vi "meas02a.vi"() -> ()   [LabVIEW 2015]
uses:
  <vilib>/DAQmx/write.llb/DAQmx Write (Analog Wfm 1Chan NSamp).vi
  <vilib>/DAQmx/create/channels.llb/DAQmx Create Channel (AO-Voltage-Basic).vi
  <vilib>/DAQmx/configure/timing.llb/DAQmx Timing (Sample Clock).vi
  <vilib>/measure/macond.llb/FIR Filter for 1 Chan.vi
  <vilib>/DAQmx/miscellaneous.llb/DAQmx Fill In Error Info.vi
  <vilib>/DAQmx/create/channels.llb/DAQmx Create Channel (CO-Pulse Generation-Frequency).vi
  <vilib>/DAQmx/configure/timing.llb/DAQmx Timing (Implicit).vi
  <vilib>/Utility/file.llb/Write Delimited Spreadsheet (DBL).vi
  <vilib>/measure/NI_MABase.lvlib
  <vilib>/measure/NI_MAPro.lvlib
panel:
  in  "Vertical Coupling (1: DC)":i32(ring)=1 items=["AC", "DC", "Ground"]
  out "Waveform Data":waveform(dbl)(graph)
  out "Log-Log Frequency and Gain":cluster{"Y":dbl[], "Y":dbl[]}[](graph)
  out "freq in":dbl
  out "Loop #":i32
  out "detected amplitude":dbl format="%.2p"
  out "detected frequency":dbl format="%.2p"
  in  "Trigger Level (0.0 V)":dbl
  in  "Trigger Mode (0: Auto)":i32(ring) items=["Auto", "Normal"]
  in  "VISA resource name":refnum<visa-resource-name>
  in  "# Points":dbl
  in  "Highest Freq":dbl
  in  "Lowest Freq":dbl
  in  "Frequency (Hz)":dbl
  in  "Stop Clock":bool
  in  "Run":bool
  in  "stop":bool
  in  "physical channels":tag
  out "Amplitude":dbl
  in  "Amplitude":dbl(knob) scale=0.0..5.0
  in  "signal type":T1(ring)
  # "Clock"
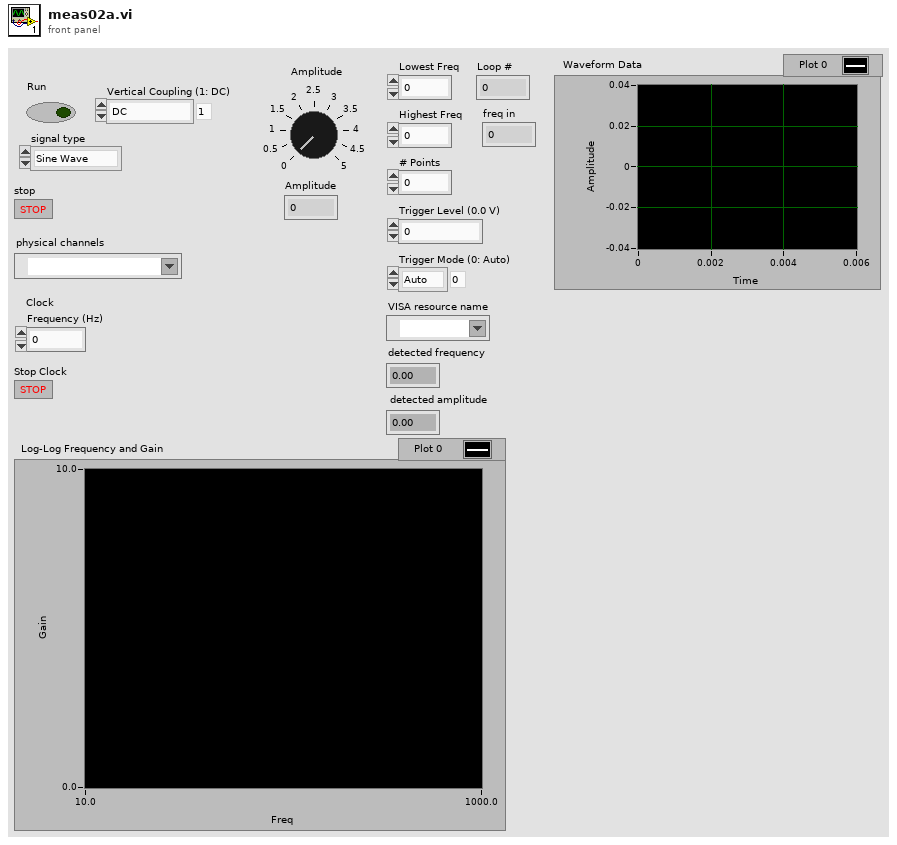
[diagram p1: front panel]
types:
  T1 = enum16{"Sine Wave", "Triangle Wave", "Square Wave", "Sawtooth Wave"}
  T2 = cluster{"Topology":enum16{"Off", "FIR by Specification", "Equi-ripple FIR", "Windowed FIR"}, "Type":enum16{"Lowpass", "Highpass", "Bandpass", "Bandstop"}, "#Taps":i32, "Lower PB":dbl, "Upper PB":dbl, "Lower SB":dbl, "Upper SB":dbl}
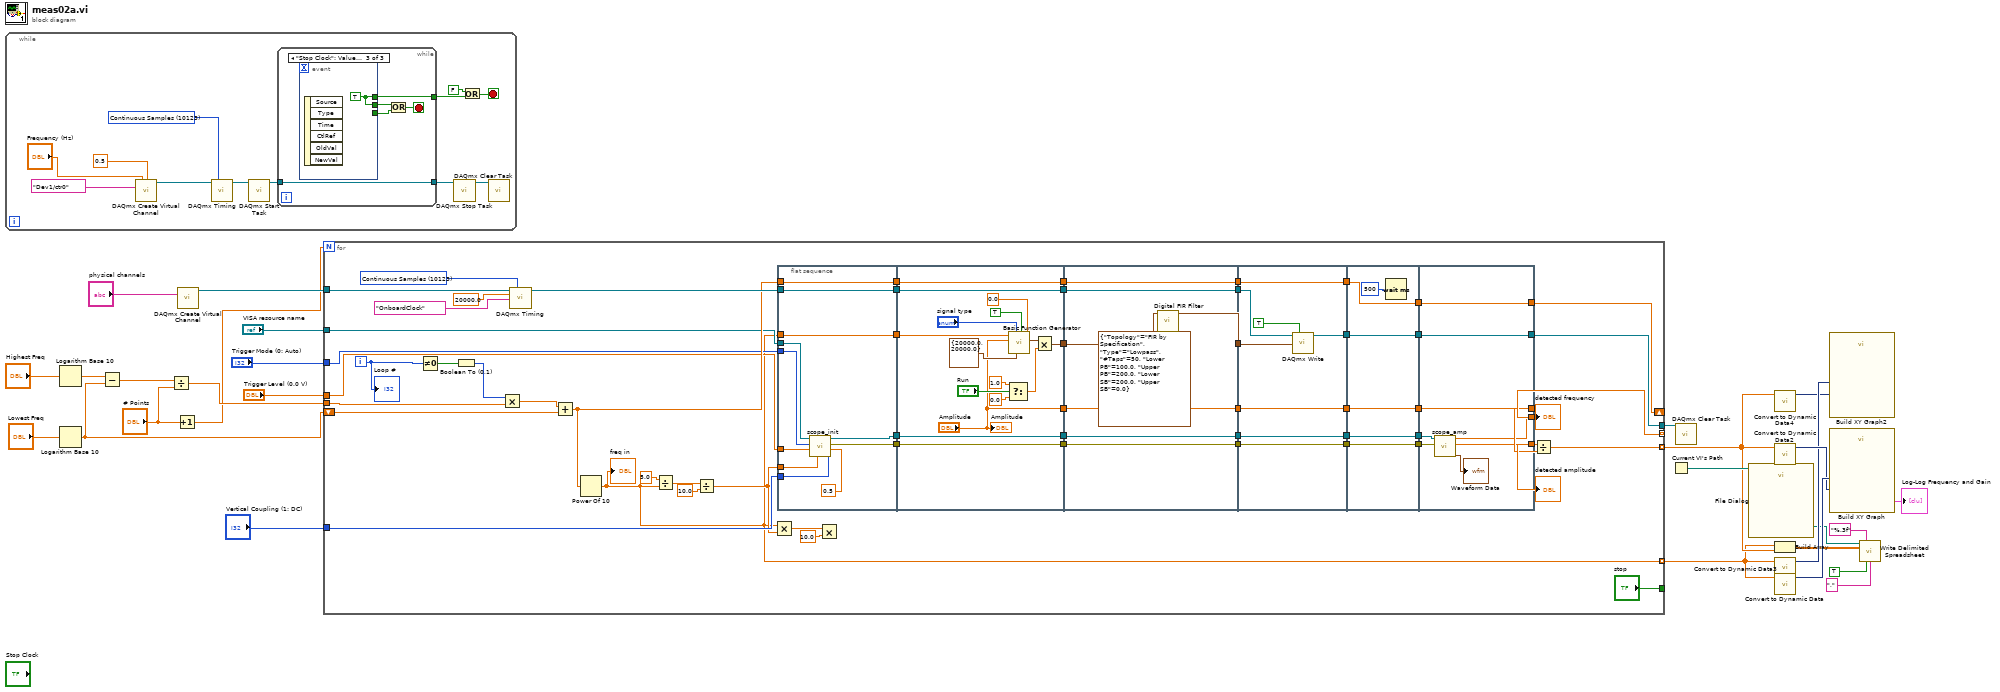
[diagram p0: block diagram]
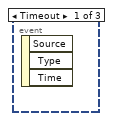
[diagram p2: hidden frame]
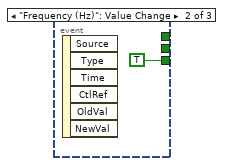
[diagram p3: hidden frame]
diagram:
  n1 = while {
    stop <- w32 stop-if-true
    w38 = 10123 items=["Finite Samples"=10178, "Continuous Samples"=10123, "Hardware Timed Single Point"=12522] ("sample mode")
    n2 = call-poly <vilib>:"DAQmx Create Virtual Channel.vi"("frequency"="Frequency (Hz)", "duty cycle"=0.5, "counter"=tag "Dev1/ctr0") -> ("task out"=w37:refnum<k21>)  [unwired: 11 in, 1 out]
    n3 = call-poly <vilib>:"DAQmx Timing.vi"("task/channels in"=w37, "sample mode"=w38) -> ("task out"=w36:refnum<k21>)  [unwired: 12 in, 1 out]
    n4 = call <vilib>:"DAQmx Start Task.vi"("task/channels in"=w36) -> ("task out"=w35:refnum<k21>)  [unwired: 13 in, 1 out]
    n5 = while {
      tunnel: w35 -> [w45]
      tunnel: [w45] -> w34
      tunnel: [w41] -> w31
      stop <- w42 stop-if-true
      n6 = event shown="[2] \"Stop Clock\": Value Change" {
        selector: _ -> [_ _ _]
        dyn-events: _ -> [_ _ _]
        timeout: _ -> [_ _ _]
        tunnel: [_ TRUE _] -> w43
        tunnel: [_ _ w47] -> w44
        tunnel: [_ _ w47] -> w41
        event Timeout {
          n7 = event-data() -> ()  [unwired: 1 in, 3 out]
        }
        event "Frequency (Hz)": Value Change {
          n8 = event-data() -> ()  [unwired: 1 in, 6 out]
        }
        event "Stop Clock": Value Change {
          w47 = TRUE
          n9 = event-data() -> ()  [unwired: 1 in, 6 out]
        }
      }
      n10 = Or(x=w44, y=w43) -> (x .or. y?=w42:bool)
    }
    n11 = call <vilib>:"DAQmx Stop Task.vi"("task/channels in"=w34) -> ("task out"=w33:refnum<k21>)  [unwired: 13 in, 1 out]
    n12 = Or(x=FALSE, y=w31) -> (x .or. y?=w32:bool)
    n13 = call <vilib>:"DAQmx Clear Task.vi"("task in"=w33) -> ()  [unwired: 14 in, 1 out]
  }
  n14 = Logarithm Base 10(1:"Highest Freq") -> (0:w20:dbl)
  n15 = Logarithm Base 10(1:"Lowest Freq") -> (0:w22:dbl)
  n16 = Subtract(x=w20, y=w22) -> (x-y=w24:dbl)
  n17 = Divide(x=w24, y="# Points") -> (x/y=w25:dbl)
  n18 = Increment(x="# Points") -> (x+1=w18:dbl)
  n19 = call-poly <vilib>:"DAQmx Create Virtual Channel.vi"("physical channels"="physical channels") -> ("task out"=w28:refnum<k21>)  [unwired: 13 in, 1 out]
  n20 = for {
    N: w18 -> [_]
    tunnel: w28 -> [w103]
    tunnel: [w80] -> w27
    tunnel: ["stop"] -> _
    tunnel: w25 -> [w98]
    tunnel: [w96] -> w2 mode=indexing
    tunnel: [w91] -> _ mode=indexing
    shift-right: [w72] -> _
    shift-left: w22 -> [w95]
    tunnel: "Trigger Level (0.0 V)" -> [w65]
    tunnel: "Trigger Mode (0: Auto)" -> [w67]
    tunnel: "VISA resource name" -> [w66]
    tunnel: "Vertical Coupling (1: DC)" -> [w64]
    tunnel: [w60] -> w1 mode=indexing
    i -> [w93]
    w100 = 10123 items=["Finite Samples"=10178, "Continuous Samples"=10123, "Hardware Timed Single Point"=12522] ("sample mode")
    n21 = Not Equal To 0?(x=w93) -> (x != 0?=w94:bool)
    n22 = Boolean To (0,1)(Boolean=w94) -> (0, 1=w92:i16)
    n23 = Multiply(x=w92, y=w98) -> (x*y=w97:dbl)
    n24 = call-poly <vilib>:"DAQmx Timing.vi"("task/channels in"=w103, "sample mode"=w100, "rate"=20000.0, "source"=tag "OnboardClock") -> ("task out"=w101:refnum<k21>)  [unwired: 10 in, 1 out]
    n25 = Add(x=w97, y=w95) -> (x+y=w73:dbl)
    n26 = Power Of 10(x=w73) -> (10^x=w60:dbl)
    "freq in" <- w60
    n27 = Divide(x=5.0, y=w60) -> (x/y=w84:dbl)
    n28 = Divide(x=w84, y=10.0) -> (x/y=w63:dbl)
    n29 = Multiply(x=w60, y=w63) -> (x*y=w62:dbl)
    n30 = flat-sequence {
      tunnel: w101 -> [w115]
      tunnel: [w115] -> w79
      tunnel: [w112] -> w78
      tunnel: [w111] -> w77
      tunnel: [w114] -> w74
      tunnel: w73 -> [w114]
      tunnel: [w113] -> w68
      tunnel: w60 -> [w113]
      tunnel: w67 -> [w107]
      tunnel: w66 -> [w110]
      tunnel: w65 -> [w108]
      tunnel: w63 -> [w109]
      tunnel: w64 -> [w105]
      tunnel: [w131] -> w59
      tunnel: [w130] -> w57
      tunnel: [w129] -> w55
      tunnel: w79 -> [w131]
      tunnel: w78 -> [w130]
      tunnel: w77 -> [w129]
      tunnel: [w128] -> w53
      tunnel: w74 -> [w128]
      tunnel: ["Amplitude"] -> w51
      tunnel: w68 -> [w127]
      tunnel: [w125] -> w49
      tunnel: w59 -> [w139]
      tunnel: [w139] -> w58
      tunnel: w57 -> [w138]
      tunnel: [w138] -> w56
      tunnel: w55 -> [w137]
      tunnel: [w137] -> w54
      tunnel: w53 -> [w136]
      tunnel: [w136] -> w52
      tunnel: w51 -> [w135]
      tunnel: [w135] -> w50
      tunnel: w49 -> [w134]
      tunnel: [w133] -> w48
      tunnel: [w146] -> w89
      tunnel: [w145] -> w87
      tunnel: [w144] -> w81
      tunnel: w58 -> [w147]
      tunnel: w56 -> [w146]
      tunnel: w54 -> [w145]
      tunnel: [w143] -> w75
      tunnel: w52 -> [w143]
      tunnel: [w142] -> w70
      tunnel: w50 -> [w142]
      tunnel: w48 -> [w140]
      tunnel: w89 -> [w153]
      tunnel: [w153] -> w88
      tunnel: w87 -> [w152]
      tunnel: [w152] -> w86
      tunnel: [w150] -> w82
      tunnel: w81 -> [w150]
      tunnel: [w149] -> w76
      tunnel: w75 -> [w149]
      tunnel: [w148] -> w71
      tunnel: w70 -> [w148]
      tunnel: w88 -> [w161]
      tunnel: w86 -> [w160]
      tunnel: [w159] -> w91
      tunnel: [w158] -> w90
      tunnel: [w157] -> w80
      tunnel: w82 -> [w157]
      tunnel: [w156] -> w72
      tunnel: w76 -> [w156]
      tunnel: [w155] -> w69
      tunnel: w71 -> [w155]
      frame #0 {
        n31 = call "scope_init.vi"("Vertical Coupling (1: DC)"=w105, "Vertical Range (10.0 V/div)"=0.5, "Timebase (0.0005 s)"=w109, "Trigger Level (0.0 V)"=w108, "Trigger Mode (0: Auto)"=w107, "VISA resource name"=w110) -> ("error out"=w111:errorcluster, "VISA resource name out"=w112:refnum<visa-resource-name>)  [unwired: 4 in]
      }
      frame #1 {
        n32 = Select(t=1.0, s="Run", f=0.0) -> (s? t:f=w121:dbl)
        n33 = call <vilib>:"Basic Function Generator.vi"("offset"=0.0, "reset signal"=TRUE, "sampling info"=cluster{"Fs":dbl, "#s":dbl} {"Fs"=20000.0, "#s"=20000.0}, "signal type"="signal type", "amplitude"="Amplitude", "frequency"=w127) -> ("signal out"=w126:waveform(dbl))  [unwired: 3 in, 2 out]
        n34 = Multiply(x=w126, y=w121) -> (x*y=w125:waveform(dbl))
        "Amplitude" <- "Amplitude"
      }
      frame #2 {
        n35 = call-poly <vilib>:"Digital FIR Filter.vi"("FIR filter specifications"=T2 {"Topology"=enum."FIR by Specification", "Type"=enum."Lowpass", "#Taps"=50, "Lower PB"=100.0, "Upper PB"=200.0, "Lower SB"=200.0, "Upper SB"=0.0}, "signal in"=w134) -> ("signal out"=w133:waveform(dbl))  [unwired: 7 in, 2 out]
      }
      frame #3 {
        n36 = call-poly <vilib>:"DAQmx Write.vi"("task/channels in"=w147, "auto start"=TRUE, "data"=w140) -> ("task out"=w144:refnum<k21>)  [unwired: 10 in, 2 out]
      }
      frame #4 {
        n37 = Wait (ms)(milliseconds to wait=u32 500) -> ()  [unwired: 1 out]
      }
      frame #5 {
        n38 = call "scope_amp.vi"("error in (no error)"=w160, "VISA resource name"=w161) -> ("Waveform Data"=→"Waveform Data":waveform(dbl), "detected amplitude"=w158:dbl, "detected frequency"=w159:dbl)  [unwired: 6 in, 1 out]
      }
    }
    n39 = Multiply(x=w62, y=10.0) -> ()  [unwired: 1 out]
    n40 = Divide(x=w90, y=w69) -> (x/y=w96:dbl)
    "detected frequency" <- w91
    "detected amplitude" <- w90
    "Loop #" <- w93
  }
  n41 = Current VI's Path() -> (path=w9:path)
  n42 = call <vilib>:"DAQmx Clear Task.vi"("task in"=w27) -> ()  [unwired: 14 in, 1 out]
  n43 = call "File Dialog"("start path"=w9) -> ("selected path"=w7:path)  [unwired: 11 in, 3 out]
  n44 = call "Convert to Dynamic Data4"("Array"=w2) -> ("Dynamic Data Type"=w13:dynamicdata)  [unwired: 3 in]
  n45 = call "Convert to Dynamic Data2"("Array"=w2) -> ("Dynamic Data Type"=w15:dynamicdata)  [unwired: 3 in]
  n46 = Build Array(w1, w2) -> (w4:dbl[][])
  n47 = call "Convert to Dynamic Data3"("Array"=w1) -> ("Dynamic Data Type"=w14:dynamicdata)  [unwired: 3 in]
  n48 = call "Convert to Dynamic Data"("Array"=w1) -> ("Dynamic Data Type"=w16:dynamicdata)  [unwired: 3 in]
  n49 = call "Build XY Graph2"("Y Input"=w13, "X Input"=w14) -> ()  [unwired: 8 in, 2 out]
  n50 = call "Build XY Graph"("Y Input"=w15, "X Input"=w16) -> ("XY Graph"=→"Log-Log Frequency and Gain":cluster{"X":dbl[], "Y":dbl[]}[])  [unwired: 8 in, 1 out]
  n51 = call-poly <vilib>:"Write Delimited Spreadsheet.vi"("file path (dialog if empty)"=w7, "format (%.3f)"="%.3f", "2D data"=w4, "transpose? (F)"=TRUE ("transpose? (no:F)"), "delimiter (\\t)"="," ("delimiter (\\t)")) -> ()  [unwired: 9 in, 2 out]
